vi "Filter the Data Frame.vi"(8 "error in (no error)":errorcluster, 11 "FE FF Frame in":refnum<class "FE FF Frame.lvclass">) -> (0 "error out":errorcluster, 3 "FE FF Frame out":refnum<class "FE FF Frame.lvclass">)   [LabVIEW 2023, in "Data Analysis.lvlib" / "FE FF Frame.lvlib" / "FE FF Frame.lvclass"]
uses:
  FE FF Frame.lvclass
  FE FF Frame.lvclass/FE FF Frame.ctl
  Data Analysis.lvlib
  HardwareAbstractionLayer_LVOOP/Database/Database.lvclass
  <vilib>/Utility/miscctls.llb/LVRowAndColumnUnsignedTypeDef.ctl
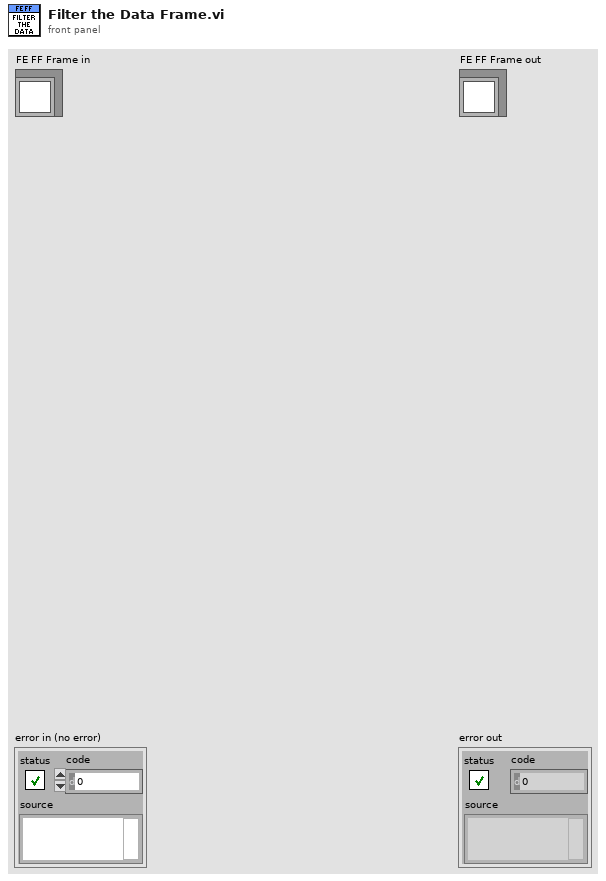
[diagram p1: front panel]
types:
  T1 = typedef "LVRowAndColumnUnsignedTypeDef.ctl" = cluster{"Row":u32, "Column":u32}
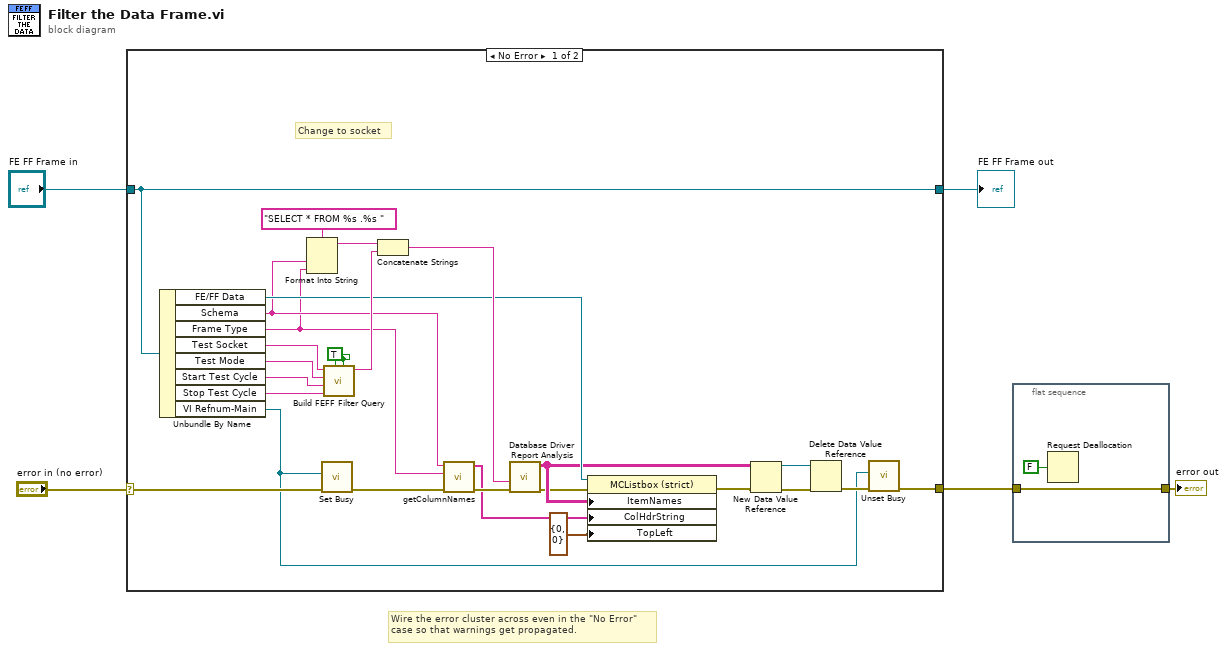
[diagram p0: block diagram]
diagram:
  # "Wire the error cluster across even in the \"No Error\"\ncase so that warnings get propagated."
  n1 = case shown="No Error" "error in (no error)" {
    selector: "error in (no error)" -> [w13 w33]
    tunnel: [w10 w33] -> w2
    tunnel: [w24 w32] -> w3
    tunnel: "FE FF Frame in" -> [w24 w32]
    frame No Error {
      w8 = TRUE ("WHERE needed?(Yes)")
      # "Change to socket"
      n2 = Unbundle By Name(w24) -> ("FE/FF Data"=w25:refnum<vi>, "Schema"=w23:string, "Frame Type"=w19:string, "Test Socket"=w22:string, "Test Mode"=w21:string, "Start Test Cycle"=w7:string, "Stop Test Cycle"=w20:string, "VI Refnum-Main"=w9:refnum<vi>)
      n3 = Format Into String(format string="SELECT * FROM %s .%s " ("SQL query"), w23, w19) -> (resulting string=w31:string)  [unwired: 2 in, 1 out]
      n4 = call <vilib>:"Set Busy.vi"("error in (no error)"=w13, "VI reference (current VI)"=w9) -> ("error out"=w12:errorcluster)  [unwired: 8 in, 1 out]
      n5 = call "Build FEFF Filter Query.vi"("ORDER BY needed?(Yes)"=w8, "WHERE needed?(Yes)"=w8, "Stop Test Cycle"=w20, "Start Test Cycle"=w7, "Test Mode"=w21, "Test Socket"=w22) -> ("String"=w28:string)  [unwired: 5 in]
      n6 = Concatenate Strings(w31, w28) -> (w29:string)
      n7 = call "getColumnNames.vi"("error in (no error)"=w12, "tableName"=w19, "schema"=w23) -> ("error out"=w27:errorcluster, "columnNames"=w26:string[])  [unwired: 6 in, 1 out]
      n8 = call "Database Driver Report Analysis.vi"("error in"=w27, "SQL query"=w29) -> ("error out"=w16:errorcluster, "data"=w18:string[][])  [unwired: 6 in, 2 out]
      n9 = property class="MCListbox (strict)"(reference=w25, error in=w16, "ItemNames"=w18, "ColHdrString"=w26, "TopLeft"=T1 {"Row"=0, "Column"=0} ("Top Left Visible Cell")) -> (error out=w15:errorcluster)  [unwired: 1 out]
      n10 = New Data Value Reference(data value=w18, error in=w15) -> (data value reference=w17:refnum<data-value>, error out=w14:errorcluster)
      n11 = Delete Data Value Reference(data value reference=w17, error in=w14) -> (error out=w11:errorcluster)  [unwired: 1 out]
      n12 = call <vilib>:"Unset Busy.vi"("error in (no error)"=w11, "VI reference (current VI)"=w9) -> ("error out"=w10:errorcluster)  [unwired: 9 in]
    }
    frame Error {
    }
  }
  "FE FF Frame out" <- w3
  n13 = flat-sequence {
    tunnel: w2 -> [w35]
    tunnel: [w35] -> w1
    frame #0 {
      n14 = Request Deallocation(FALSE ("flag")) -> ()
    }
  }
  "error out" <- w1
